vi "Write.vi"(8 "error in":errorcluster, 10 "ICommunicate":refnum<class "ICommunicate.lvclass">, 11 "CANopen Message in":refnum<class "CANopen Message.lvclass">) -> (0 "error out":errorcluster, 3 "CANopen Message out":refnum<class "CANopen Message.lvclass">)   [LabVIEW 2024, in "CANopen Master.lvlib" / "CANopen Message.lvclass"]
uses:
  CANopen Message.lvclass
  HAL/Source/Interfaces/ICommunicate/ICommunicate.lvclass
  CANopen Message.lvclass/CANopen Message.ctl
  HAL/Source/Messages/CAN Message/CAN Message.lvclass
  D:/git/HAL/Source/Messages/CAN Message/CAN Message.lvclass
  D:/git/HAL/Source/Interfaces/IMessage/IMessage.lvclass
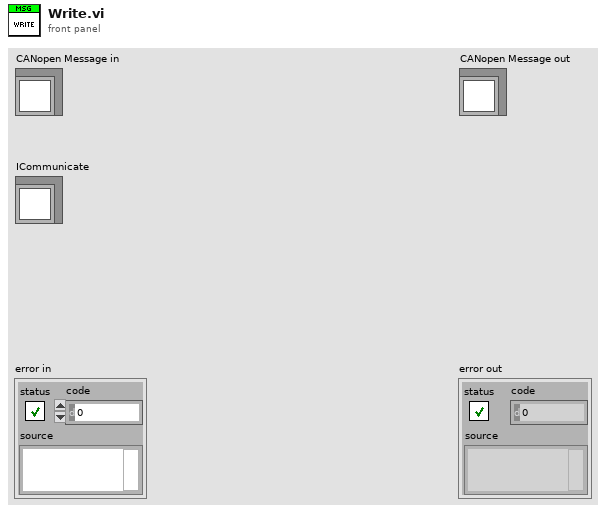
[diagram p1: front panel]
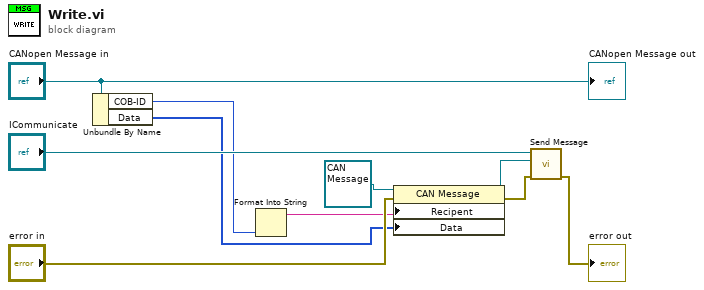
[diagram p0: block diagram]
diagram:
  n1 = Unbundle By Name("CANopen Message in") -> ("COB-ID"=w3:u32, "Data"=w5:u8[])
  n2 = Format Into String(w3) -> (resulting string=w4:string)  [unwired: 3 in, 1 out]
  n3 = property class="CAN Message"(reference=refnum<class "CAN Message.lvclass"> refnum ("CAN Message"), error in="error in", "Recipent"=w4, "Data"=w5) -> (reference out=w2:refnum<class "CAN Message.lvclass">, error out=w6:errorcluster)
  n4 = call-dynamic "Send Message.vi"("error in"=w6, "IMessage"=w2, "ICommunicate in"="ICommunicate") -> ("error out"=→"error out":errorcluster)  [unwired: 7 in, 1 out]
  "CANopen Message out" <- "CANopen Message in"
